vi "New Connection MHLC.vi"(8 "error in (no error)":errorcluster, 10 "Data in":variant, 11 "TCPServer in":refnum<class "DS TCP Server.lvclass">) -> (0 "error out":errorcluster, 3 "TCPServer out":refnum<class "DS TCP Server.lvclass">)   [LabVIEW 2017, in "DS TCP Server.lvlib" / "DS TCP Server.lvclass"]
doc: "A new connection has been established to a Debug Client. Verify that the Debug Client is UID is valid. If YES, then create a TCP Read Worker to handle the incoming data to the Debug Client."
uses:
  DS TCP Server.lvclass
  rsp_Incompatible DC Connection.ctl
  <vilib>/addons/_Workers/Library/Classes/Message/Priority.ctl
  Connection ID.ctl
  Common VIs/DC_UID.ctl
  rql_Create Read Worker.ctl
  <vilib>/addons/_Workers/Library/Classes/Message Queue/Message Queue.lvclass
  DS TCP Server.lvclass/DS TCP Server.ctl
  <vilib>/Utility/error.llb/Error Cluster From Error Code.vi
  <vilib>/ErrorRing/Error Ring.xnode
  DS TCP Listener/DS TCP Listener.lvclass
  <vilib>/addons/_Workers/Library/Classes/Message/Message.lvclass
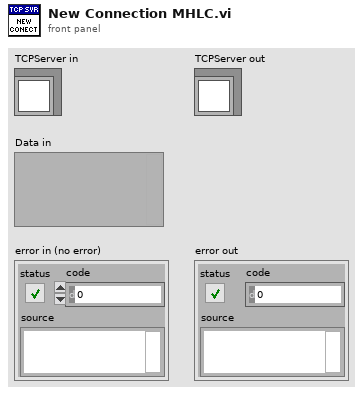
[diagram p1: front panel]
types:
  T1 = typedef "DS TCP Server.lvlib/DS TCP Listener.lvclass/rsp_New Connection.ctl" = cluster{"Connection Ref":refnum<k5>, "Name":string, "Message Priority":T2, "IP Address":string}
  T2 = typedef "Workers.lvlib/Message.lvclass/Priority.ctl" = enum16{"Low", "Normal", "High"}
  T3 = typedef "DS TCP Server.lvlib/DS TCP Server.lvclass/rsp_Incompatible DC Connection.ctl" = cluster{"DC Version":string, "IP Address":string}
  T4 = typedef "DS TCP Server.lvlib/DS TCP Server.lvclass/rql_Create Read Worker.ctl" = cluster{"Forwarding Q":refnum<class "Message Queue.lvclass">, "DC_UID":T5, "Worker Alias":string, "Message Priority":T2}
  T5 = typedef "DC_UID.ctl" = string
  T6 = typedef "DS TCP Server.lvlib/DS TCP Server.lvclass/Connection ID.ctl" = cluster{"Connection Ref":refnum<k5>, "DC_UID":T5, "Message Priority":T2, "IP Address":string}
  T7 = typedef "DS TCP Server.lvlib/DS TCP Server.lvclass/Message Log Data.ctl" = cluster{"Message Log Q":refnum<class "Message Queue.lvclass">, "Message Log ID":T8, "DC_UID":T5}
  T8 = typedef "Message Log ID.ctl" = cluster{"Head Worker ID":string, "IP Address":string}
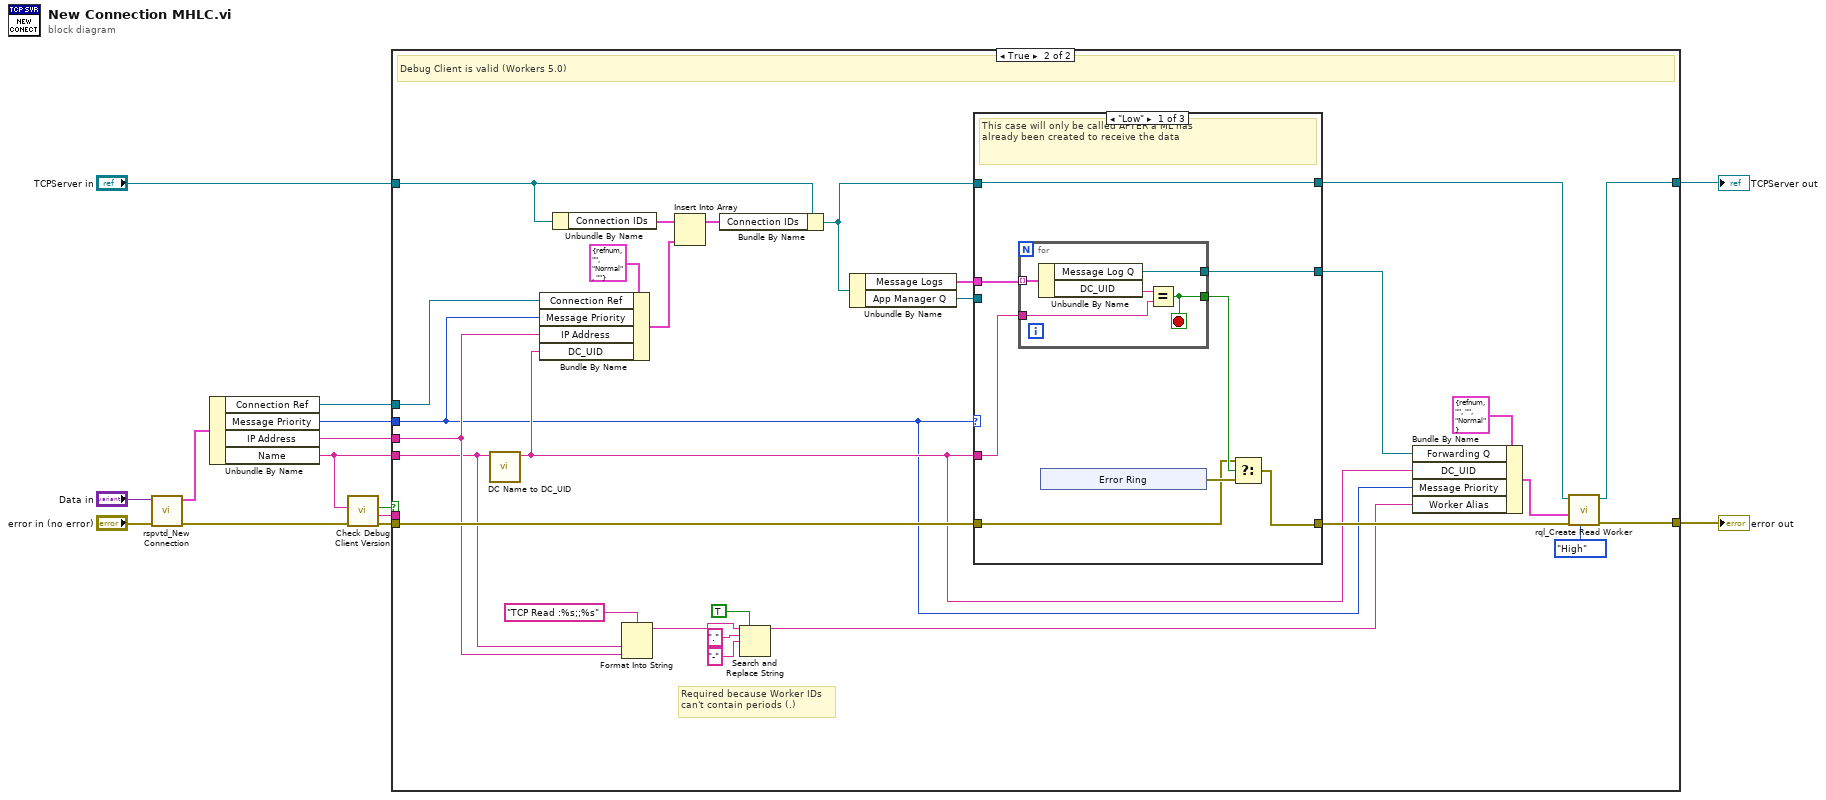
[diagram p0: block diagram]
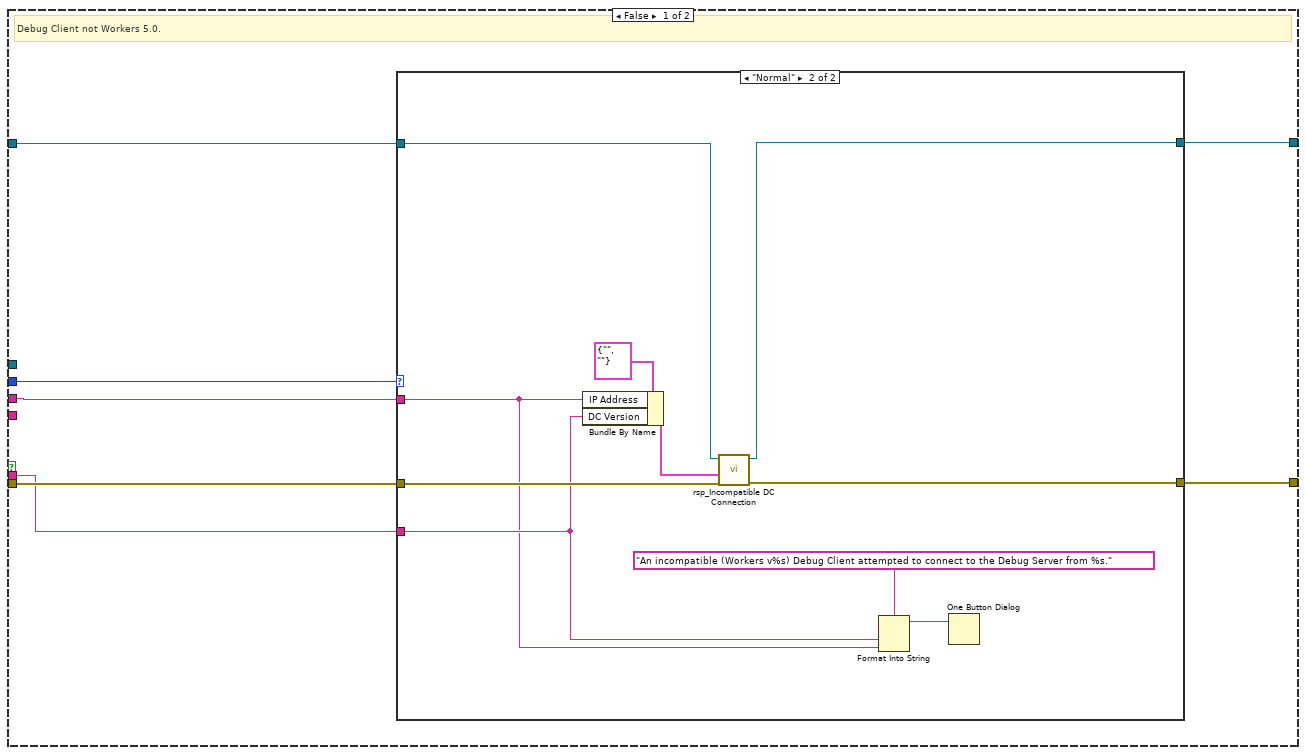
[diagram p2: hidden frame]
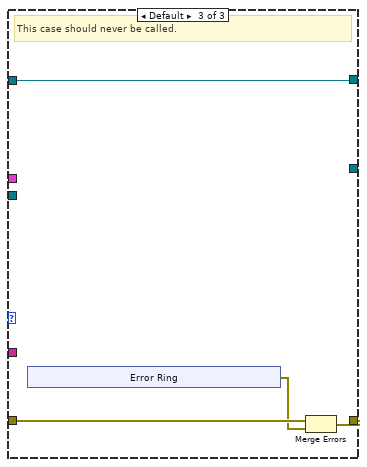
[diagram p5: hidden frame]
diagram:
  n1 = call "rspvtd_New Connection.vi"("error in"="error in (no error)", "Data in"="Data in") -> ("error out"=w12:errorcluster, "Data out"=w10:T1)  [unwired: 8 in]
  n2 = Unbundle By Name(w10) -> ("Connection Ref"=w11:refnum<k5>, "Message Priority"=w6:T2, "IP Address"=w9:string, "Name"=w4:string)
  n3 = call "Check Debug Client Version.vi"("error in (no error)"=w12, "Debug Client Name"=w4) -> ("error out"=w5:errorcluster, "DC Version"=w1:string, "Valid"=w2:bool)  [unwired: 7 in]
  n4 = case shown="True" w2 {
    tunnel: "TCPServer in" -> [w19 w61]
    tunnel: w5 -> [w21 w52]
    tunnel: w11 -> [_ w50]
    tunnel: w9 -> [w16 w47]
    tunnel: w4 -> [_ w34]
    tunnel: [w20 w40] -> w8
    tunnel: [w18 w39] -> w7
    tunnel: w6 -> [w15 w36]
    tunnel: w1 -> [w17 _]
    frame False {
      # "Debug Client not Workers 5.0."
      n5 = case shown="\"Normal\"" w15 {
        tunnel: w21 -> [w23 w33]
        tunnel: [w23 w32] -> w20
        tunnel: w19 -> [w22 w31]
        tunnel: [w22 w30] -> w18
        tunnel: w17 -> [_ w26]
        tunnel: w16 -> [_ w25]
        frame Default {
        }
        frame "Normal" {
          n6 = Bundle By Name(cluster=T3 {"DC Version"="", "IP Address"=""} ("Data in"), "IP Address"=w25, "DC Version"=w26) -> (w28:T3)
          n7 = call "rsp_Incompatible DC Connection.vi"("error in"=w33, "Data in"=w28, "DS TCP Server in"=w31) -> ("error out"=w32:errorcluster, "dup DS TCP Server out"=w30:refnum<class "DS TCP Server.lvclass">)  [unwired: 7 in]
          n8 = Format Into String(format string="An incompatible (Workers v%s) Debug Client attempted to connect to the Debug Server from %s." ("message"), w26, w25) -> (resulting string=w24:string)  [unwired: 2 in, 1 out]
          n9 = One Button Dialog(message=w24) -> ()  [unwired: 1 in, 1 out]
        }
      }
    }
    frame True {
      # "Required because Worker IDs\ncan't contain periods (.)"
      # "Debug Client is valid (Workers 5.0)"
      n10 = call "DC Name to DC_UID.vi"("DC Name"=w34) -> ("DC_UID"=w37:T5)  [unwired: 10 in]
      n11 = Bundle By Name(cluster=T6 {"Connection Ref"=refnum, "DC_UID"="", "Message Priority"=enum."Normal", "IP Address"=""} ("new element/subarray"), "Connection Ref"=w50, "Message Priority"=w36, "IP Address"=w47, "DC_UID"=w37) -> (w49:T6)
      n12 = Unbundle By Name(w61) -> ("Connection IDs"=w60:T6[])
      n13 = Format Into String(format string="TCP Read :%s;;%s" ("Worker Alias"), w34, w47) -> (resulting string=w54:string)  [unwired: 2 in, 1 out]
      n14 = Insert Into Array(array=w60, new element=w49) -> (w59:T6[])  [unwired: 1 in]
      n15 = Bundle By Name(cluster=w61, "Connection IDs"=w59) -> (w48:refnum<class "DS TCP Server.lvclass">)
      n16 = Search and Replace String(replace all?=TRUE ("replace all? (F)"), input string=w54, search string=".", replace string="-" ("replace string (\"\")")) -> (result string=w35:string)  [unwired: 4 in, 3 out]
      n17 = Unbundle By Name(w48) -> ("Message Logs"=w46:T7[], "App Manager Q"=w53:refnum<class "Message Queue.lvclass">)
      n18 = case shown="\"Low\"" w36 {
        tunnel: w53 -> [_ w80 _]
        tunnel: w52 -> [w65 w82 w86]
        tunnel: [w63 w82 w85] -> w41
        tunnel: w48 -> [w62 w81 w83]
        tunnel: [w62 w81 w83] -> w38
        tunnel: w46 -> [w69 _ _]
        tunnel: w37 -> [w68 _ _]
        tunnel: [w64 w80 _] -> w42
        frame "Low" {
          # "This case will only be called AFTER a ML has \nalready been created to receive the data"
          n19 = for {
            tunnel: w69 -> [w79] mode=indexing
            tunnel: w68 -> [w77]
            tunnel: [w76] -> w66
            tunnel: [w75] -> w64
            stop <- w76 stop-if-true
            n20 = Unbundle By Name(w79) -> ("Message Log Q"=w75:refnum<class "Message Queue.lvclass">, "DC_UID"=w78:T5)
            n21 = Equal?(x=w78, y=w77) -> (x = y?=w76:bool)
          }
          n22 = xnode "Error Ring"() -> ("error out"=w67:errorcluster)
          n23 = Select(t=w65, s=w66, f=w67) -> (s? t:f=w63:errorcluster)
        }
        frame "Normal" {
          # "Normal priority. Nothing to do."
        }
        frame Default {
          # "This case should never be called."
          n24 = xnode "Error Ring"() -> ("error out"=w84:errorcluster)
          n25 = Merge Errors(w86, w84) -> (w85:errorcluster)
        }
      }
      n26 = Bundle By Name(cluster=T4 {"Forwarding Q"=refnum, "DC_UID"="", "Worker Alias"="", "Message Priority"=enum."Normal"} ("Data in"), "Forwarding Q"=w42, "DC_UID"=w37, "Message Priority"=w36, "Worker Alias"=w35) -> (w45:T4)
      n27 = call "rql_Create Read Worker.vi"("Message Priority"=Priority."High", "error in"=w41, "Data in"=w45, "DS TCP Server in"=w38) -> ("error out"=w40:errorcluster, "dup DS TCP Server out"=w39:refnum<class "DS TCP Server.lvclass">)  [unwired: 6 in]
    }
  }
  "error out" <- w8
  "TCPServer out" <- w7
